vi "Pre Launch Init.vi"(11 "Data Repository in":refnum<class "Data Repository.lvclass">) -> (0 "error out":errorcluster, 3 "Data Repository out":refnum<class "Data Repository.lvclass">)   [LabVIEW 2020, in "Data Repository.lvlib" / "Data Repository.lvclass"]
doc: "(<B>Filename</B>: Actor Framework.lvlib:Actor.lvclass:Pre Launch Init.vi)\n\nDefines behavior that occurs after the Launch Nested Actor method is invoked but before the actor's Actor Core method begins running.\n\nThis implementation sets up a subscription for Data messages."
uses:
  Data Repository.lvclass
  PPL/HDH.Actor Framework.Core.Actor.lvlibp/1abvi3w/vi.lib/ActorFramework/Message Enqueuer/Message Priority.ctl
  PPL/HDH.Actor Framework.Core.Publisher.lvlibp/Messages/Data Msg/Data Msg.lvclass
  C:/Current projects/WS/PPL/HDH.Actor Framework.Core.Actor.lvlibp/1abvi3w/vi.lib/ActorFramework/Message/Message.lvclass
  PPL/HDH.Actor Framework.Core.Actor.lvlibp/1abvi3w/vi.lib/ActorFramework/Actor/Actor.lvclass
  PPL/HDH.Actor Framework.Core.Publisher.lvlibp/Publisher Messages/Subscribe Msg/Subscribe Msg.lvclass
  PPL/HDH.Actor Framework.Core.Actor.lvlibp/1abvi3w/vi.lib/ActorFramework/Message Enqueuer/Message Enqueuer.lvclass
  C:/Current projects/WS/PPL/HDH.Actor Framework.Core.Actor.lvlibp/1abvi3w/vi.lib/ActorFramework/Actor/Actor.lvclass
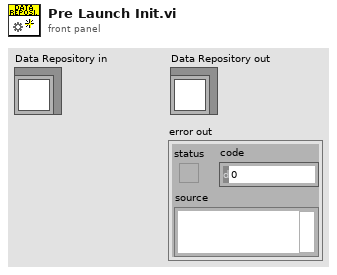
[diagram p1: front panel]
types:
  T1 = typedef "HDH.Actor Framework.Core.Actor.lvlibp/Message Enqueuer.lvclass/Message Priority.ctl" = enum16{"Low", "Normal", "High"}
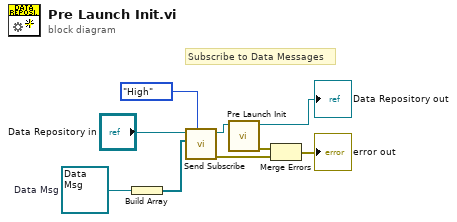
[diagram p0: block diagram]
diagram:
  w7 = refnum<class "Data Msg.lvclass"> refnum  # Data Msg
  # "Subscribe to Data Messages"
  n1 = Build Array(w7) -> (w6:refnum<class "Data Msg.lvclass">[])
  n2 = call "Send Subscribe.vi"("Message Priority (High)"=Message_Priority."High", "Message Array"=w6, "Actor in"="Data Repository in") -> ("error out"=w1:errorcluster, "Actor out"=w3:refnum<class "Data Repository.lvclass">)  [unwired: 7 in]
  n3 = call-parent "Pre Launch Init.vi"("Actor in"=w3) -> ("error out"=w9:errorcluster, "Actor out"=→"Data Repository out":refnum<class "Data Repository.lvclass">)  [unwired: 9 in]
  n4 = Merge Errors(w9, w1) -> (→"error out":errorcluster)
